vi "Keithley 6517A Single Read Example2.vi"(0 "GPIB address":string="1:27", 1 "function (Vdc:0)":u16(ring)=1 items=["dc voltage", "dc current", "resistance", "charge"], 3 "error in":T1) -> (4 "units":string="ADC", 5 "reading #":dbl=1.0, 6 "measurement":dbl=3.26757e-12 format="%.6e", 7 "time and date stamp":string="03:56:41.00,15-Jul-  94", 9 "error out":T1)   [LabVIEW 2013]
doc: "This EXAMPLE VI takes a single reading. The data returned includes the reading, timestamp, units, and reading#. Since this is an example, you are free to alter the VI to add addtional elements. Adding or deleting elements will requiore you to modify the VI to separate all of the elements into their individual components."
panel:
  out "?":string="+03.26757E-12ADC,03:56:41.00,15-Jul-  94,+00001RDNG#\n"
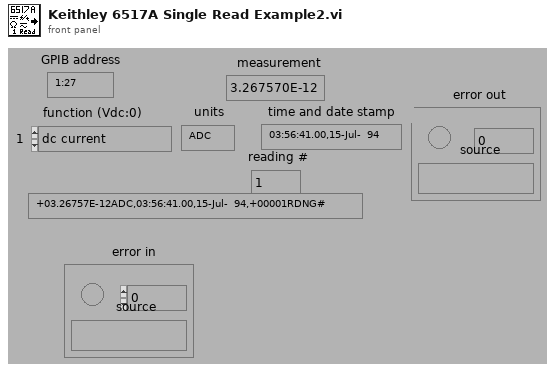
[diagram p1: front panel]
types:
  T1 = cluster{"error":bool, "code":i32, "source":string}
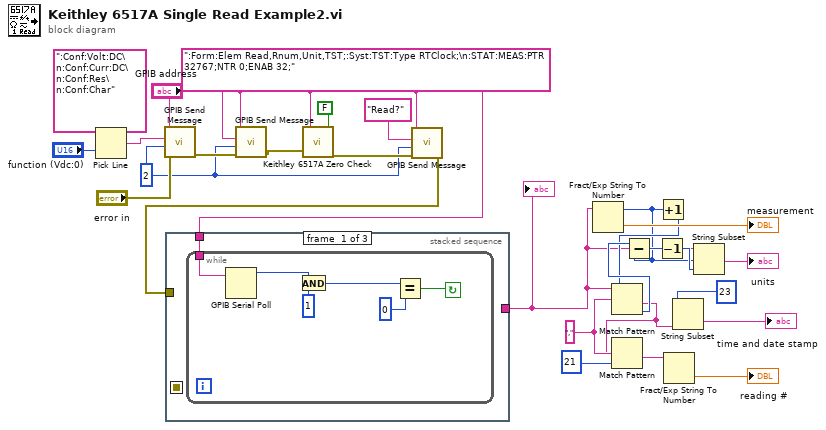
[diagram p0: block diagram]
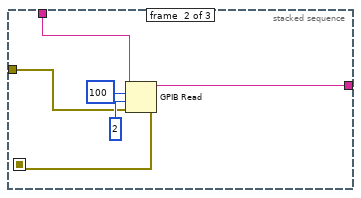
[diagram p2: hidden frame]
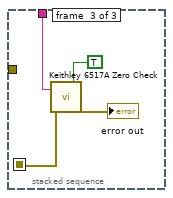
[diagram p3: hidden frame]
diagram:
  w25 = ","
  w4 = 2
  n1 = Pick Line(multi-line string=":Conf:Volt:DC\n:Conf:Curr:DC\n:Conf:Res\n:Conf:Char", line index="function (Vdc:0)") -> (output string=w11:string)  [unwired: 1 in]
  n2 = call "GPIB Send Message.vi"("address string"="GPIB address", "write buffer"=w11, "write mode (set END:0)"=w4, "error in"="error in") -> ("error out"=w9:T1)  [unwired: 3 in, 2 out]
  n3 = call "GPIB Send Message.vi"("address string"="GPIB address", "write buffer"=":Form:Elem Read,Rnum,Unit,TST;:Syst:TST:Type RTClock;\n:STAT:MEAS:PTR 32767;NTR 0;ENAB 32;", "write mode (set END:0)"=w4, "error in"=w9) -> ("error out"=w7:T1)  [unwired: 3 in, 2 out]
  n4 = call "Keithley 6517A Zero Check.vi"("Zero Check"=FALSE, "error in"=w7, "GPIB address"="GPIB address") -> ("error out"=w6:T1)
  n5 = call "GPIB Send Message.vi"("address string"="GPIB address", "write buffer"="Read?", "write mode (set END:0)"=w4, "error in"=w6) -> ("error out"=w3:T1)  [unwired: 3 in, 2 out]
  n6 = stacked-sequence {
    seq-local: [_ w39 _] -> [_ _ w44]
    tunnel: [_ w41 _] -> w1
    tunnel: w3 -> [_ w37 _]
    tunnel: "GPIB address" -> [w29 w36 w42]
    frame #0 {
      n7 = while {
        tunnel: w29 -> [w30]
        stop <- w34 continue-if-true
        n8 = GPIB Serial Poll(0:w30) -> (2:w33:i16)  [unwired: 1 in, 2 out]
        n9 = And(x=w33, y=1) -> (x .and. y?=w31:i32)
        n10 = Equal?(x=w31, y=0) -> (x = y?=w34:bool)
      }
    }
    frame #1 {
      n11 = GPIB Read(0:w36, 1:100, 2:2, 3:w37) -> (5:w41:string, 7:w39:errorcluster)  [unwired: 1 in, 1 out]
    }
    frame #2 {
      n12 = call "Keithley 6517A Zero Check.vi"("Zero Check"=TRUE, "error in"=w44, "GPIB address"=w42) -> ("error out"=→"error out":T1)
    }
  }
  "?" <- w1
  n13 = Fract/Exp String To Number(string=w1) -> (offset past number=w15:i32, number=→"measurement":dbl)  [unwired: 3 in]
  n14 = Increment(x=w15) -> (x+1=w16:i32)
  n15 = Match Pattern(string=w1, regular expression=w25, offset (0)=w16) -> (after substring=w19:string, offset past match=w23:i32)  [unwired: 2 out]
  n16 = Match Pattern(string=w19, regular expression=w25, offset (0)=21) -> (after substring=w24:string)  [unwired: 3 out]
  n17 = Subtract(x=w23, y=w15) -> (x-y=w21:i32)
  n18 = Decrement(x=w21) -> (x-1=w22:i32)
  n19 = Fract/Exp String To Number(string=w24) -> (number=→"reading #":dbl)  [unwired: 3 in, 1 out]
  n20 = String Subset(string=w19, length (rest)=23) -> (substring=→"time and date stamp":string)  [unwired: 1 in]
  n21 = String Subset(string=w1, offset (0)=w15, length (rest)=w22) -> (substring=→"units":string)
